vi "Colors Read.vi"(4 "error in (no error)":errorcluster, 6 "Container State":T5, 7 "Display State In":T2={"Draw Options"={"Outer Border Color"=0, "Inner Border Color"=6316128, "Outer Gradient Color"=2565927, "Inner Gradient Color"=16860, "Compass North Pointer Color"=16711680, "Compass Pointer Color 1"=13355429, "Compass Pointer Color 2"=14934973, "Direction Pointer Color"=16765184, "Text Box Outline Color"=13355429, "Text Box Background Color"=14934973, "Scale Color"=16448250, "Text Color"=0, "Draw Gradient"=TRUE, "Draw Rose"=TRUE, "Simple Scale"=TRUE, "Draw Text"=FALSE, "Font Name"="Helvetica", "Angle Units"=enum."Degrees"}}) -> (0 "error out":errorcluster, 2 "Value":T1={"Outer Border Color"=0, "Inner Border Color"=6316128, "Outer Gradient Color"=2565927, "Inner Gradient Color"=16860, "Compass North Pointer Color"=16711680, "Compass Pointer Color 1"=13355429, "Compass Pointer Color 2"=14934973, "Direction Pointer Color"=16765184, "Text Box Outline Color"=13355429, "Text Box Background Color"=14934973, "Scale Color"=16448250, "Text Color"=0}, 3 "Display State Out":T2={"Draw Options"={"Outer Border Color"=0, "Inner Border Color"=6316128, "Outer Gradient Color"=2565927, "Inner Gradient Color"=16860, "Compass North Pointer Color"=16711680, "Compass Pointer Color 1"=13355429, "Compass Pointer Color 2"=14934973, "Direction Pointer Color"=16765184, "Text Box Outline Color"=13355429, "Text Box Background Color"=14934973, "Scale Color"=16448250, "Text Color"=0, "Draw Gradient"=TRUE, "Draw Rose"=TRUE, "Simple Scale"=TRUE, "Draw Text"=FALSE, "Font Name"="Helvetica", "Angle Units"=enum."Degrees"}})   [LabVIEW 2017, in "Compass Indicator.xctl"]
uses:
  <vilib>/robotics/Controls/Compass Indicator/Compass Indicator.xctl
  <vilib>/_xctls/Container State.ctl
  <vilib>/robotics/Controls/Compass Indicator/_Compass Indicator Support Files/Compass State.ctl
  <vilib>/robotics/Controls/Compass Indicator/Compass Picture/Draw Options.ctl
  <vilib>/robotics/Controls/Utilities/Angle Units.ctl
  <vilib>/_xctls/XControlSupport.lvlib
  <vilib>/robotics/Controls/Compass Indicator/Compass Picture/NI_Robotics_Compass Picture.lvlib
  <vilib>/robotics/Controls/Utilities/NI_Robotics_Control Utilities.lvlib
panel:
  # "Replace the Value Indicator below with an Indicator of desired type.\nDo not remove this Indicator or the others from the connector pane. \nDo not change the connector pane pattern.\nThe Value Indicator should always be the second terminal from top on the output side in the connector pane."
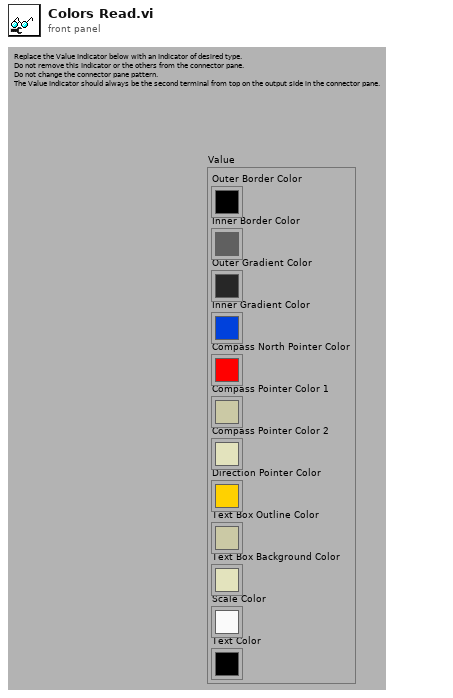
[diagram p1: front panel]
types:
  T1 = cluster{"Outer Border Color":u32, "Inner Border Color":u32, "Outer Gradient Color":u32, "Inner Gradient Color":u32, "Compass North Pointer Color":u32, "Compass Pointer Color 1":u32, "Compass Pointer Color 2":u32, "Direction Pointer Color":u32, "Text Box Outline Color":u32, "Text Box Background Color":u32, "Scale Color":u32, "Text Color":u32}
  T2 = typedef "Compass Indicator.xctl/Compass State.ctl" = cluster{"Draw Options":T3}
  T3 = typedef "NI_Robotics_Compass Picture.lvlib/Draw Options.ctl" = cluster{"Outer Border Color":u32, "Inner Border Color":u32, "Outer Gradient Color":u32, "Inner Gradient Color":u32, "Compass North Pointer Color":u32, "Compass Pointer Color 1":u32, "Compass Pointer Color 2":u32, "Direction Pointer Color":u32, "Text Box Outline Color":u32, "Text Box Background Color":u32, "Scale Color":u32, "Text Color":u32, "Draw Gradient":bool, "Draw Rose":bool, "Simple Scale":bool, "Draw Text":bool, "Font Name":string, "Angle Units":T4}
  T4 = typedef "NI_Robotics_Control Utilities.lvlib/Angle Units.ctl" = enum16{"Radians", "Degrees"}
  T5 = typedef "XControlSupport.lvlib/Container State.ctl" = cluster{"Indicator?":bool, "Run Mode?":bool, " Refnum":refnum<vi>}
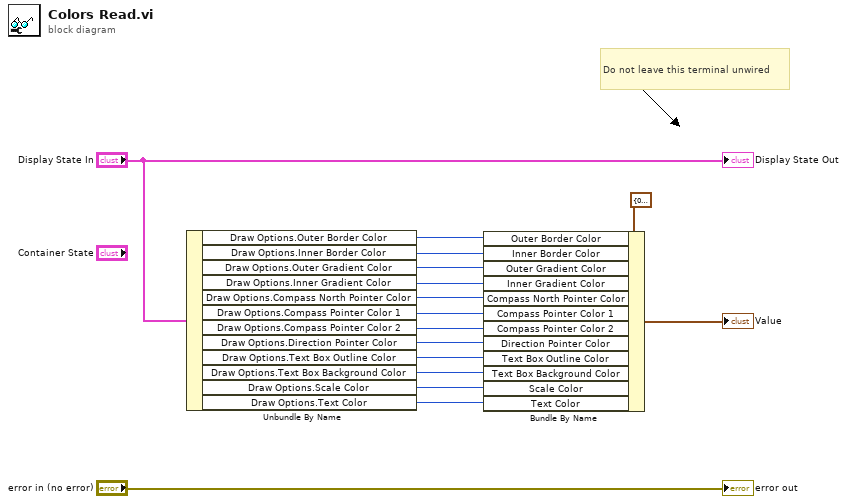
[diagram p0: block diagram]
diagram:
  # "Do not leave this terminal unwired"
  n1 = Unbundle By Name("Display State In") -> ("Draw Options.Outer Border Color"=w13:u32, "Draw Options.Inner Border Color"=w12:u32, "Draw Options.Outer Gradient Color"=w11:u32, "Draw Options.Inner Gradient Color"=w10:u32, "Draw Options.Compass North Pointer Color"=w9:u32, "Draw Options.Compass Pointer Color 1"=w8:u32, "Draw Options.Compass Pointer Color 2"=w7:u32, "Draw Options.Direction Pointer Color"=w6:u32, "Draw Options.Text Box Outline Color"=w5:u32, "Draw Options.Text Box Background Color"=w4:u32, "Draw Options.Scale Color"=w3:u32, "Draw Options.Text Color"=w2:u32)
  n2 = Bundle By Name(cluster=T1 {"Outer Border Color"=0, "Inner Border Color"=0, "Outer Gradient Color"=0, "Inner Gradient Color"=0, "Compass North Pointer Color"=0, "Compass Pointer Color 1"=0, "Compass Pointer Color 2"=0, "Direction Pointer Color"=0, "Text Box Outline Color"=0, "Text Box Background Color"=0, "Scale Color"=0, "Text Color"=0} ("Value"), "Outer Border Color"=w13, "Inner Border Color"=w12, "Outer Gradient Color"=w11, "Inner Gradient Color"=w10, "Compass North Pointer Color"=w9, "Compass Pointer Color 1"=w8, "Compass Pointer Color 2"=w7, "Direction Pointer Color"=w6, "Text Box Outline Color"=w5, "Text Box Background Color"=w4, "Scale Color"=w3, "Text Color"=w2) -> (→"Value":T1)
  "error out" <- "error in (no error)"
  "Display State Out" <- "Display State In"
